vi "Tempo&TrigSARAH.vi"(4 "entrée d'erreur (pas d'erreur)":errorcluster, 5 "Tempo Mes-Largage (ms)":u32=3000, 6 "Tempo Houle - Mes (ms)":u32=3000, 7 "task in":refnum<k21>) -> (0 "sortie d'erreur":errorcluster)   [LabVIEW 2017]
uses:
  DefDeType/MachEtatStartSARAH.ctl
  <vilib>/DAQmx/write.llb/DAQmx Write (Digital Bool 1Line 1Point).vi
  <vilib>/DAQmx/read.llb/DAQmx Read (Digital Bool 1Line 1Point).vi
  <vilib>/DAQmx/create/channels.llb/DAQmx Create Channel (DI-Digital Input).vi
  <vilib>/DAQmx/create/channels.llb/DAQmx Create Channel (DO-Digital Output).vi
  <vilib>/DAQmx/miscellaneous.llb/DAQmx Fill In Error Info.vi
panel:
  out "Trig Largueur":bool
  out "Trig Mesures":bool
  out "Info":string
  in  "Bouton Annuler":bool
  out "Tempo 2":u32(slide) scale=0.0..1000.0
  out "Tempo 1":u32(slide) scale=0.0..5000.0
  out "iteration":i32
  out "Trig Batteur":bool
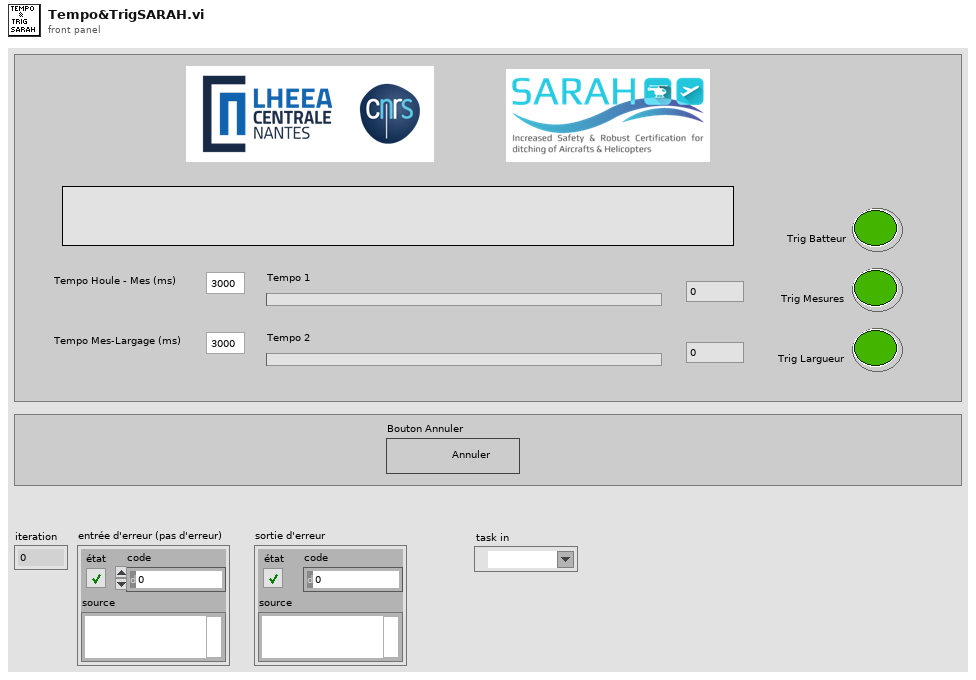
[diagram p1: front panel]
types:
  T1 = typedef "MachEtatStartSARAH.ctl" = enum16{"AttenteTrigBatteur", "TempoHoule-Mes", "TempoMes-Largage", "Quitter"}
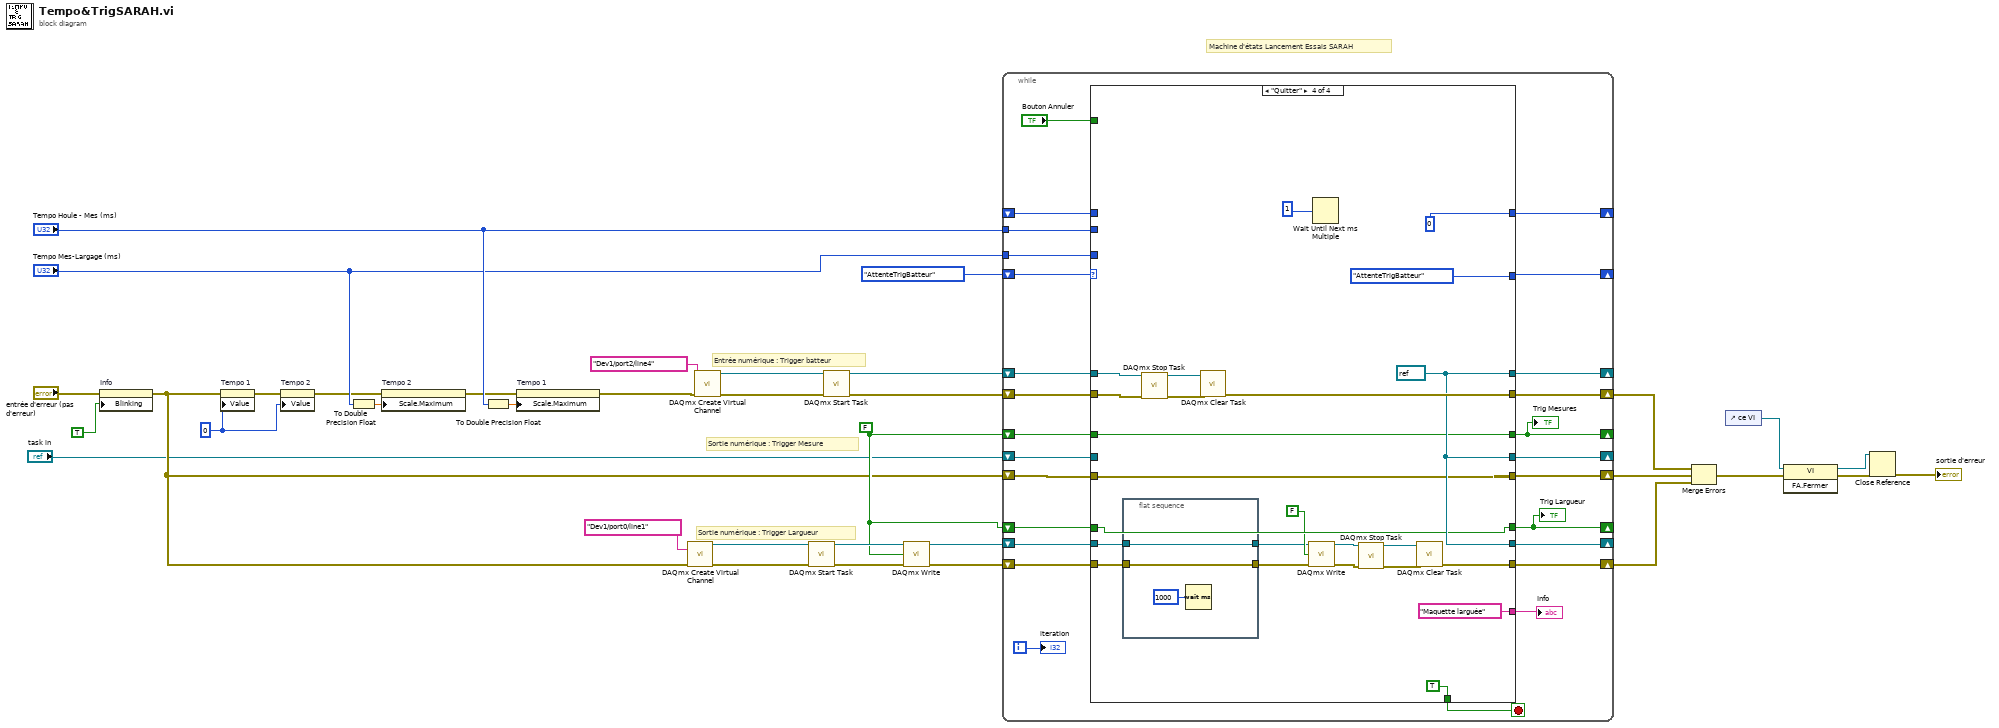
[diagram p0: block diagram]
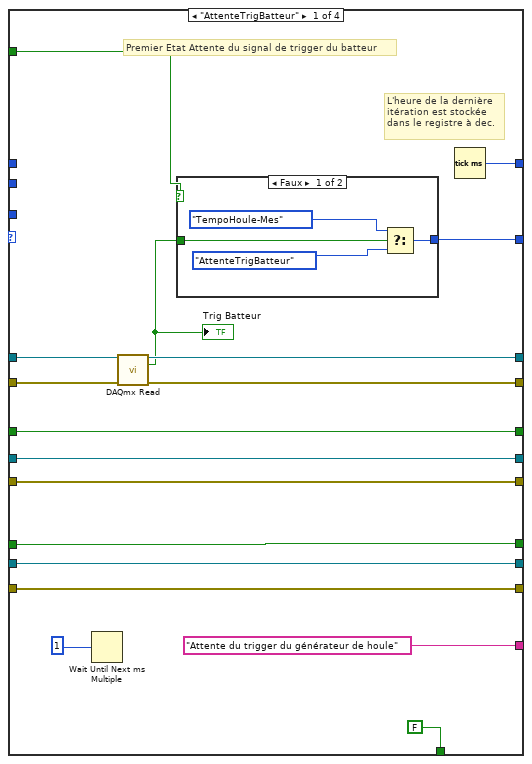
[diagram p2: hidden frame]
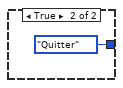
[diagram p3: hidden frame]
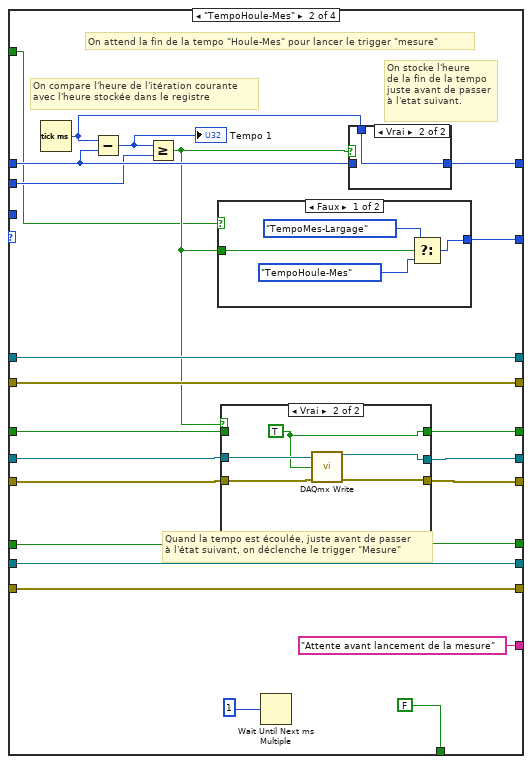
[diagram p4: hidden frame]
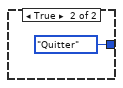
[diagram p5: hidden frame]
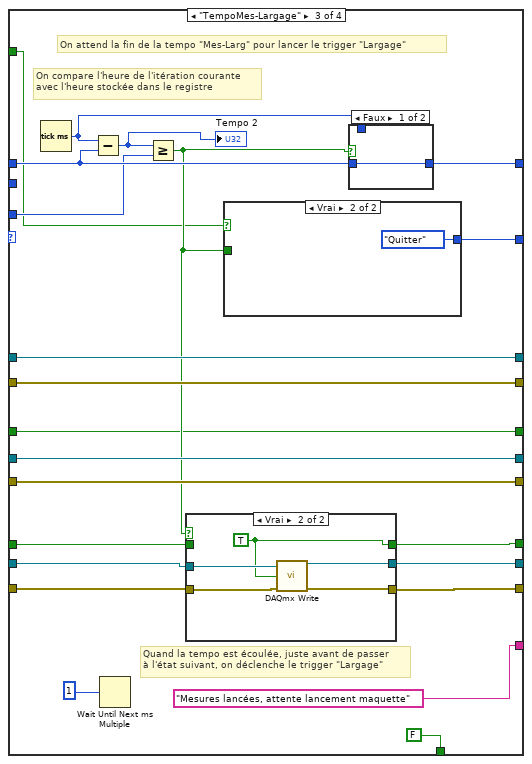
[diagram p8: hidden frame]
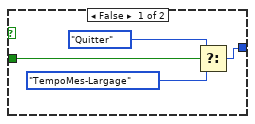
[diagram p9: hidden frame]
diagram:
  w15 = u32 0 ("Tempo 1")
  w13 = FALSE ("data")
  # "Sortie numérique : Trigger Largueur"
  # "Sortie numérique : Trigger Mesure"
  # "Entrée numérique : Trigger batteur"
  # "Machine d'états Lancement Essais SARAH"
  n1 = property on="Info" class="Ch"(error in="entrée d'erreur (pas d'erreur)", "Blinking"=TRUE ("Clignotant")) -> (error out=w2:errorcluster)  [unwired: 1 in, 1 out]
  n2 = property on="Tempo 1" class="Gliss (strict)"(error in=w2, "Value"=w15) -> (error out=w16:errorcluster)  [unwired: 1 in, 1 out]
  n3 = property on="Tempo 2" class="Gliss (strict)"(error in=w16, "Value"=w15) -> (error out=w14:errorcluster)  [unwired: 1 in, 1 out]
  n4 = To Double Precision Float(number="Tempo Mes-Largage (ms)") -> (double precision float=w18:dbl)
  n5 = property on="Tempo 2" class="Gliss (strict)"(error in=w14, "Scale.Maximum"=w18) -> (error out=w19:errorcluster)  [unwired: 1 in, 1 out]
  n6 = To Double Precision Float(number="Tempo Houle - Mes (ms)") -> (double precision float=w21:dbl)
  n7 = property on="Tempo 1" class="Gliss (strict)"(error in=w19, "Scale.Maximum"=w21) -> (error out=w22:errorcluster)  [unwired: 1 in, 1 out]
  n8 = call-poly <vilib>:"DAQmx Create Virtual Channel.vi"("lines"=tag "Dev1/port0/line1", "error in"=w2) -> ("task out"=w28:refnum<k21>, "error out"=w27:errorcluster)  [unwired: 12 in]
  n9 = call-poly <vilib>:"DAQmx Create Virtual Channel.vi"("lines"=tag "Dev1/port2/line4", "error in"=w22) -> ("task out"=w34:refnum<k21>, "error out"=w33:errorcluster)  [unwired: 12 in]
  n10 = call <vilib>:"DAQmx Start Task.vi"("task/channels in"=w28, "error in"=w27) -> ("task out"=w26:refnum<k21>, "error out"=w25:errorcluster)  [unwired: 12 in]
  n11 = call <vilib>:"DAQmx Start Task.vi"("task/channels in"=w34, "error in"=w33) -> ("task out"=w31:refnum<k21>, "error out"=w32:errorcluster)  [unwired: 12 in]
  n12 = call-poly <vilib>:"DAQmx Write.vi"("task/channels in"=w26, "data"=w13, "error in"=w25) -> ("task out"=w23:refnum<k21>, "error out"=w24:errorcluster)  [unwired: 10 in, 1 out]
  n13 = while {
    shift-right: [w57] -> _
    shift-left: MachEtatStartSARAH."AttenteTrigBatteur" -> [w53]
    shift-right: [w59] -> _
    shift-left: w31 -> [w60]
    shift-right: [w58] -> w12
    shift-left: w32 -> [w61]
    shift-right: [w55] -> _
    shift-left: _ -> [w54]
    shift-right: [w45] -> _
    shift-left: "task in" -> [w51]
    shift-right: [w47] -> w11
    shift-left: w2 -> [w50]
    shift-right: [w44] -> _
    shift-left: w23 -> [w49]
    shift-right: [w46] -> w10
    shift-left: w24 -> [w48]
    tunnel: "Tempo Houle - Mes (ms)" -> [w43]
    tunnel: "Tempo Mes-Largage (ms)" -> [w42]
    shift-right: [w38] -> _
    shift-left: w13 -> [w39]
    shift-right: [w36] -> _
    shift-left: w13 -> [w37]
    i -> [w56]
    stop <- w52 stop-if-true
    n14 = case shown="\"Quitter\"" w53 {
      tunnel: w61 -> [w78 w104 w141 w174]
      tunnel: w60 -> [w77 w105 w142 w175]
      tunnel: [w75 w105 w142 w169] -> w59
      tunnel: [w74 w104 w141 w171] -> w58
      tunnel: [w73 w102 w139 MachEtatStartSARAH."AttenteTrigBatteur"] -> w57
      tunnel: [w72 w100 w137 u32 0 ("millisecond timer value")] -> w55
      tunnel: w54 -> [_ w101 w138 _]
      tunnel: [FALSE ("stop") FALSE ("stop") FALSE ("stop") TRUE ("stop")] -> w52
      tunnel: w51 -> [w67 w96 w134 _]
      tunnel: w50 -> [w66 w95 w133 w165]
      tunnel: w49 -> [w70 w92 w132 w164]
      tunnel: w48 -> [w69 w91 w131 w163]
      tunnel: [w66 w93 w133 w165] -> w47
      tunnel: [w69 w91 w129 w170] -> w46
      tunnel: [w67 w94 w134 w169] -> w45
      tunnel: [w70 w92 w130 w169] -> w44
      tunnel: w43 -> [_ w89 _ _]
      tunnel: w42 -> [_ _ w126 _]
      tunnel: "Bouton Annuler" -> [w65 w88 w125 _]
      tunnel: ["Attente du trigger du générateur de houle" ("Info") "Attente avant lancement de la mesure" ("Info") "Mesures lancées, attente lancement maquette" ("Info") "Maquette larguée" ("Info")] -> w40
      tunnel: w39 -> [w63 w86 w123 w167]
      tunnel: [w63 w85 w123 w167] -> w38
      tunnel: [w62 w84 w121 w166] -> w36
      tunnel: w37 -> [w62 w84 w122 w166]
      frame "AttenteTrigBatteur" {
        # "L'heure de la dernière \nitération est stockée \ndans le registre à dec."
        # "Premier Etat Attente du signal de trigger du batteur"
        n15 = Wait Until Next ms Multiple(millisecond multiple=u32 1 ("attente (ms)")) -> ()  [unwired: 1 out]
        n16 = call-poly <vilib>:"DAQmx Read.vi"("task/channels in"=w77, "error in"=w78) -> ("task out"=w75:refnum<k21>, "data"=w68:bool, "error out"=w74:errorcluster)  [unwired: 11 in]
        "Trig Batteur" <- w68
        n17 = case shown="Faux" w65 {
          tunnel: [w82 MachEtatStartSARAH."Quitter"] -> w73
          tunnel: w68 -> [w79 _]
          frame False {
            n18 = Select(t=MachEtatStartSARAH."TempoHoule-Mes", s=w79, f=MachEtatStartSARAH."AttenteTrigBatteur") -> (s? t:f=w82:T1)
          }
          frame True {
          }
        }
        n19 = Tick Count (ms)() -> (millisecond timer value=w72:u32)
      }
      frame "TempoHoule-Mes" {
        # "Quand la tempo est écoulée, juste avant de passer \nà l'état suivant, on déclenche le trigger \"Mesure\""
        # "On stocke l'heure \nde la fin de la tempo\njuste avant de passer\nà l'etat suivant."
        # "On compare l'heure de l'itération courante\navec l'heure stockée dans le registre"
        # "On attend la fin de la tempo \"Houle-Mes\" pour lancer le trigger \"mesure\""
        n20 = Tick Count (ms)() -> (millisecond timer value=w99:u32)
        n21 = Subtract(x=w99, y=w101) -> (x-y=w90:u32)
        "Tempo 1" <- w90
        n22 = Greater Or Equal?(x=w90, y=w89) -> (x >= y?=w97:bool)
        n23 = case shown="Faux" w88 {
          tunnel: [w109 MachEtatStartSARAH."Quitter"] -> w102
          tunnel: w97 -> [w106 _]
          frame False {
            n24 = Select(t=MachEtatStartSARAH."TempoMes-Largage", s=w106, f=MachEtatStartSARAH."TempoHoule-Mes") -> (s? t:f=w109:T1)
          }
          frame True {
          }
        }
        n25 = case shown="Vrai" w97 {
          tunnel: [w113 w116] -> w94
          tunnel: w96 -> [w113 w118]
          tunnel: [w112 w115] -> w93
          tunnel: w95 -> [w112 w117]
          tunnel: w86 -> [w111 _]
          tunnel: [w111 w114] -> w85
          frame False {
          }
          frame True {
            w114 = TRUE ("data")
            n26 = call-poly <vilib>:"DAQmx Write.vi"("task/channels in"=w118, "data"=w114, "error in"=w117) -> ("task out"=w116:refnum<k21>, "error out"=w115:errorcluster)  [unwired: 10 in, 1 out]
          }
        }
        n27 = Wait Until Next ms Multiple(millisecond multiple=u32 1 ("attente (ms)")) -> ()  [unwired: 1 out]
        n28 = case shown="Vrai" w97 {
          tunnel: w101 -> [w119 _]
          tunnel: [w119 w120] -> w100
          tunnel: w99 -> [_ w120]
          frame False {
          }
          frame True {
          }
        }
      }
      frame "TempoMes-Largage" {
        # "Quand la tempo est écoulée, juste avant de passer \nà l'état suivant, on déclenche le trigger \"Largage\""
        # "On compare l'heure de l'itération courante\navec l'heure stockée dans le registre"
        # "On attend la fin de la tempo \"Mes-Larg\" pour lancer le trigger \"Largage\""
        n29 = Tick Count (ms)() -> (millisecond timer value=w136:u32)
        n30 = Subtract(x=w136, y=w138) -> (x-y=w127:u32)
        "Tempo 2" <- w127
        n31 = Wait Until Next ms Multiple(millisecond multiple=u32 1 ("attente (ms)")) -> ()  [unwired: 1 out]
        n32 = Greater Or Equal?(x=w127, y=w126) -> (x >= y?=w128:bool)
        n33 = case shown="Vrai" w128 {
          tunnel: [w150 w153] -> w130
          tunnel: w132 -> [w150 w155]
          tunnel: [w149 w152] -> w129
          tunnel: w131 -> [w149 w154]
          tunnel: w122 -> [w148 _]
          tunnel: [w148 w151] -> w121
          frame False {
          }
          frame True {
            w151 = TRUE ("data")
            n34 = call-poly <vilib>:"DAQmx Write.vi"("task/channels in"=w155, "data"=w151, "error in"=w154) -> ("task out"=w153:refnum<k21>, "error out"=w152:errorcluster)  [unwired: 10 in, 1 out]
          }
        }
        n35 = case shown="Vrai" w125 {
          tunnel: [w146 MachEtatStartSARAH."Quitter"] -> w139
          tunnel: w128 -> [w143 _]
          frame False {
            n36 = Select(t=MachEtatStartSARAH."Quitter", s=w143, f=MachEtatStartSARAH."TempoMes-Largage") -> (s? t:f=w146:T1)
          }
          frame True {
          }
        }
        n37 = case shown="Faux" w128 {
          tunnel: w138 -> [w156 _]
          tunnel: [w156 w157] -> w137
          tunnel: w136 -> [_ w157]
          frame False {
          }
          frame True {
          }
        }
      }
      frame "Quitter" {
        w169 = refnum<k21> refnum ("task out")
        n38 = flat-sequence {
          tunnel: w164 -> [w182]
          tunnel: w163 -> [w183]
          tunnel: [w182] -> w159
          tunnel: [w183] -> w158
          frame #0 {
            n39 = Wait (ms)(milliseconds to wait=u32 1000 ("attente (ms)")) -> ()  [unwired: 1 out]
          }
        }
        n40 = call <vilib>:"DAQmx Stop Task.vi"("task/channels in"=w175, "error in"=w174) -> ("task out"=w176:refnum<k21>, "error out"=w177:errorcluster)  [unwired: 12 in]
        n41 = call <vilib>:"DAQmx Clear Task.vi"("task in"=w176, "error in"=w177) -> ("error out"=w171:errorcluster)  [unwired: 13 in]
        n42 = call-poly <vilib>:"DAQmx Write.vi"("task/channels in"=w159, "data"=FALSE, "error in"=w158) -> ("task out"=w160:refnum<k21>, "error out"=w161:errorcluster)  [unwired: 10 in, 1 out]
        n43 = Wait Until Next ms Multiple(millisecond multiple=u32 1 ("attente (ms)")) -> ()  [unwired: 1 out]
        n44 = call <vilib>:"DAQmx Stop Task.vi"("task/channels in"=w160, "error in"=w161) -> ("task out"=w172:refnum<k21>, "error out"=w173:errorcluster)  [unwired: 12 in]
        n45 = call <vilib>:"DAQmx Clear Task.vi"("task in"=w172, "error in"=w173) -> ("error out"=w170:errorcluster)  [unwired: 13 in]
      }
    }
    "Info" <- w40
    "Trig Mesures" <- w38
    "Trig Largueur" <- w36
    "iteration" <- w56
  }
  n46 = Merge Errors(w12, w11, w10) -> (w9:errorcluster)
  n47 = control-ref of="ce VI"() -> (w8:refnum<vi>)
  n48 = invoke class="VI" method="FA.Fermer"(reference=w8, error in=w9) -> (reference out=w5:refnum<vi>, error out=w7:errorcluster)  [unwired: 1 in, 1 out]
  n49 = Close Reference(reference=w5, error in (no error)=w7) -> (error out=→"sortie d'erreur":errorcluster)
